vi "Get_Trck_Mean_Inst-t_Vel-s_Durat-n_Length-1.vi"(4 "error IN":errorcluster, 7 "[IN] Tracks + Starting Position":cluster{"Tracks":dbl[], "Start Pos":i32}[](array[cluster])) -> (0 "error OUT":errorcluster, 1 "[OUT] Track length":dbl[](array[numeric]), 2 "[OUT] Track Duration":u16[](array[numeric]), 3 "[OUT] Mean Instant Vel-s":dbl[](array[numeric]))   [LabVIEW 2013]
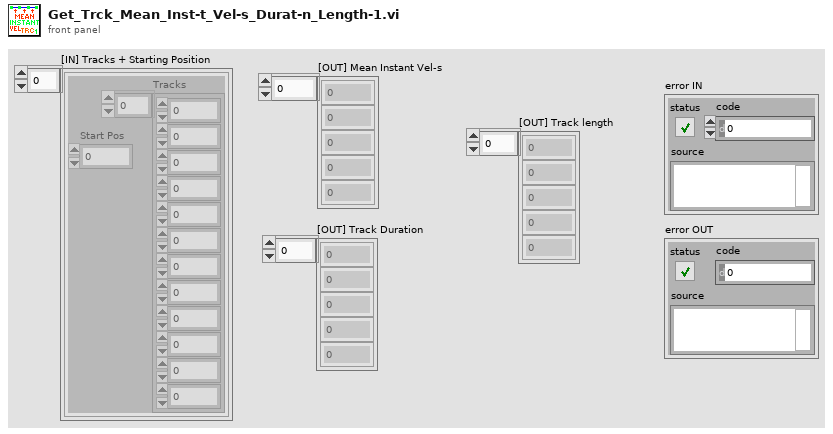
[diagram p1: front panel]
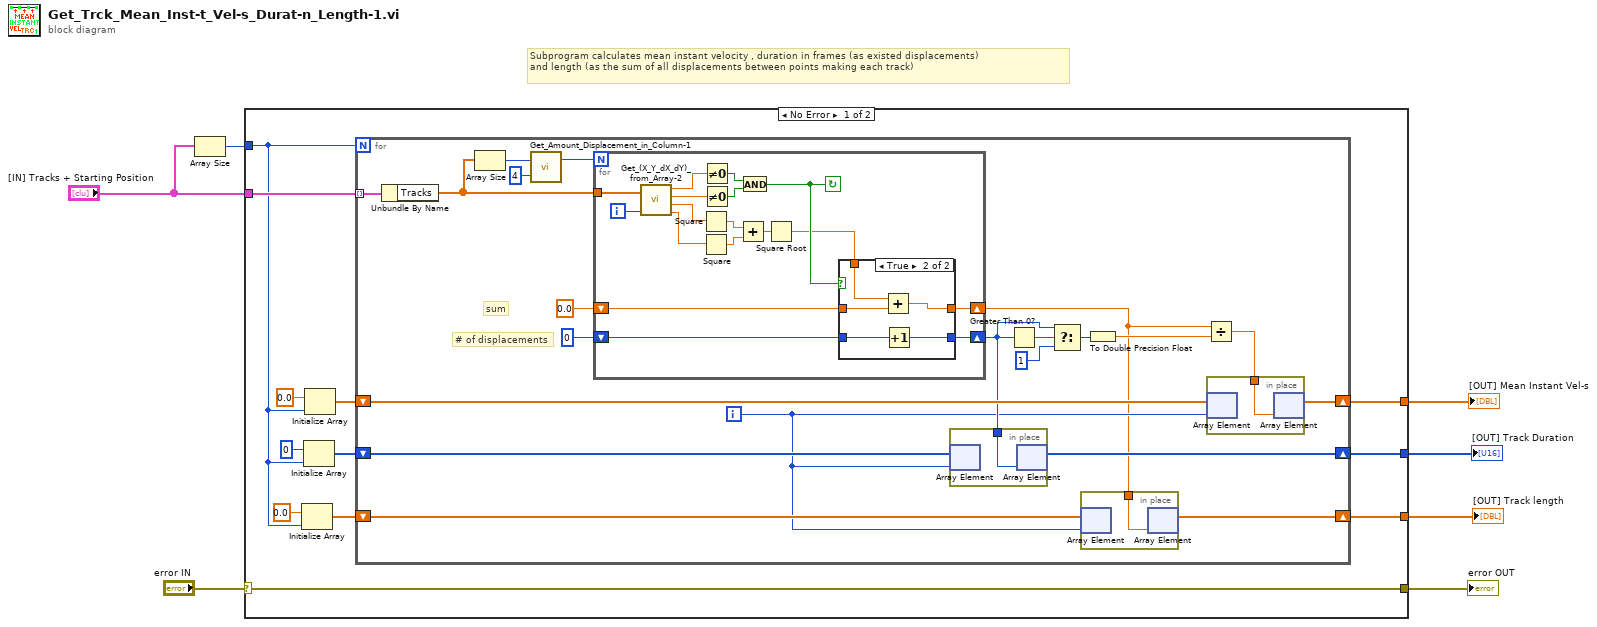
[diagram p0: block diagram]
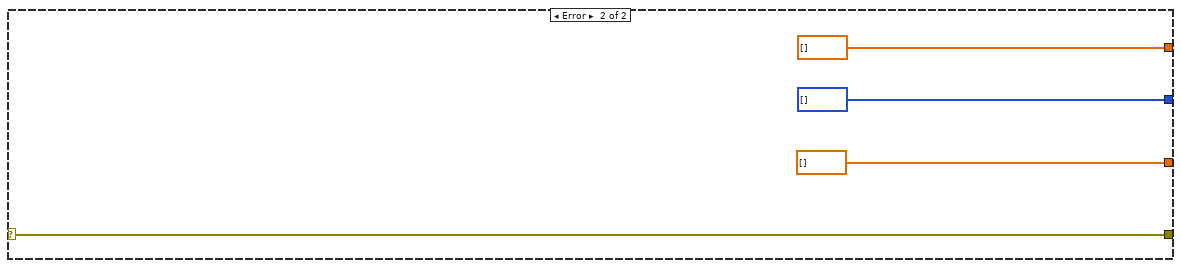
[diagram p3: hidden frame]
diagram:
  # "Subprogram calculates mean instant velocity , duration in frames (as existed displacements) \nand length (as the sum of all displacements between points making each track)"
  n1 = Array Size(array="[IN] Tracks + Starting Position") -> (size(s)=w6:i32)
  n2 = case shown="No Error" "error IN" {
    selector: "error IN" -> [w16 w70]
    tunnel: w6 -> [w10 _]
    tunnel: "[IN] Tracks + Starting Position" -> [w19 _]
    tunnel: [w16 w70] -> w4
    tunnel: [w15 dbl[] []] -> w3
    tunnel: [w12 u16[] []] -> w2
    tunnel: [w8 dbl[] []] -> w1
    frame No Error {
      n3 = Initialize Array(0.0 ("element"), w10) -> (w9:dbl[])
      n4 = Initialize Array(u16 0 ("element"), w10) -> (w13:u16[])
      n5 = Initialize Array(0.0 ("element"), w10) -> (w17:dbl[])
      n6 = for {
        N: w10 -> [_]
        tunnel: w19 -> [w40] mode=indexing
        shift-right: [w27] -> w15
        shift-left: w17 -> [w29]
        shift-right: [w24] -> w12
        shift-left: w13 -> [w26]
        shift-right: [w20] -> w8
        shift-left: w9 -> [w23]
        i -> [w22]
        # "sum"
        # "# of displacements"
        n7 = Unbundle By Name(w40) -> ("Tracks"=w36:dbl[])
        n8 = Array Size(array=w36) -> (size(s)=w38:i32)
        n9 = call "Get_Amount_Displacement_in_Column-1.vi"("multiplier"=4, "# Rows"=w38) -> ("Displ amount"=w37:i32)  [unwired: 1 out]
        n10 = for {
          N: w37 -> [_]
          tunnel: w36 -> [w59]
          shift-right: [w47] -> w25
          shift-left: u16 0 -> [w48]
          shift-right: [w44] -> w21
          shift-left: 0.0 -> [w46]
          i -> [w60]
          stop <- w49 continue-if-true
          n11 = call "Get_(X_Y_dX_dY)_from_Array-2.vi"("(X,Y,dX,dY)"=w59, "Index of Displacement"=w60) -> ("X"=w58:dbl, "Y"=w57:dbl, "dX"=w54:dbl, "dY"=w53:dbl)
          n12 = Square(x=w54) -> (x^2=w52:dbl)
          n13 = Square(x=w53) -> (x^2=w51:dbl)
          n14 = Not Equal To 0?(x=w58) -> (x != 0?=w56:bool)
          n15 = Not Equal To 0?(x=w57) -> (x != 0?=w55:bool)
          n16 = Add(x=w52, y=w51) -> (x+y=w50:dbl)
          n17 = And(x=w56, y=w55) -> (x .and. y?=w49:bool)
          n18 = Square Root(x=w50) -> (sqrt(x)=w45:dbl)
          n19 = case shown="True" w49 {
            tunnel: w48 -> [w61 w67]
            tunnel: [w61 w66] -> w47
            tunnel: w46 -> [w62 w65]
            tunnel: w45 -> [_ w64]
            tunnel: [w62 w63] -> w44
            frame False {
            }
            frame True {
              n20 = Add(x=w64, y=w65) -> (x+y=w63:dbl)
              n21 = Increment(x=w67) -> (x+1=w66:u16)
            }
          }
        }
        n22 = in-place {
          in-place-border: w25 -> [w42]
          n23 = in-place-array #1(w26, w22) -> ()  [unwired: 1 out]
          n24 = in-place-array #1(w42) -> (w24:u16[])  [unwired: 1 out]
        }
        n25 = Greater Than 0?(x=w25) -> (x > 0?=w33:bool)
        n26 = Select(t=w25, s=w33, f=u16 1) -> (s? t:f=w31:u16)
        n27 = in-place {
          in-place-border: w21 -> [w41]
          n28 = in-place-array #2(w23, w22) -> ()  [unwired: 1 out]
          n29 = in-place-array #2(w41) -> (w20:dbl[])  [unwired: 1 out]
        }
        n30 = To Double Precision Float(number=w31) -> (double precision float=w30:dbl)
        n31 = Divide(x=w21, y=w30) -> (x/y=w28:dbl)
        n32 = in-place {
          in-place-border: w28 -> [w43]
          n33 = in-place-array #3(w29, w22) -> ()  [unwired: 1 out]
          n34 = in-place-array #3(w43) -> (w27:dbl[])  [unwired: 1 out]
        }
      }
    }
    frame Error {
    }
  }
  "error OUT" <- w4
  "[OUT] Mean Instant Vel-s" <- w3
  "[OUT] Track Duration" <- w2
  "[OUT] Track length" <- w1
